vi "禹山pH_获取温度和测量值.vi"(8 "error in (no error)":errorcluster caption="错误输入（无错误）", 11 "MB_Serial session in":refnum<class "MB_Master_Serial.lvclass">) -> (0 "error out":errorcluster caption="错误输出", 2 "输出值":cluster{"温度测量值":sgl, "ORP":sgl, "pH":sgl}, 3 "MB_Serial session out":refnum<class "MB_Master_Serial.lvclass">)   [LabVIEW 2016, in "斯坦道多参数.lvlib"]
uses:
  <vilib>/Plasmionique/MB Master/MB_Master_Serial/MB_Master_Serial.lvclass
  C:/Program Files (x86)/National Instruments/LabVIEW 2016/vi.lib/Plasmionique/MB Master/MB_Master/MB_Master.lvclass
  <vilib>/Plasmionique/MB Master/MB Master.lvlib
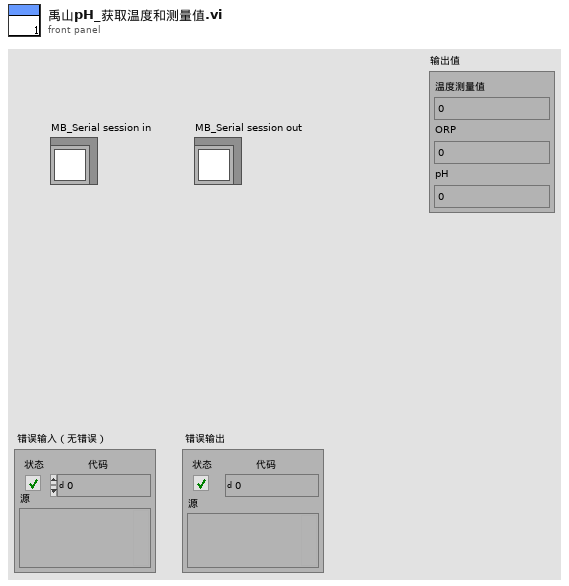
[diagram p1: front panel]
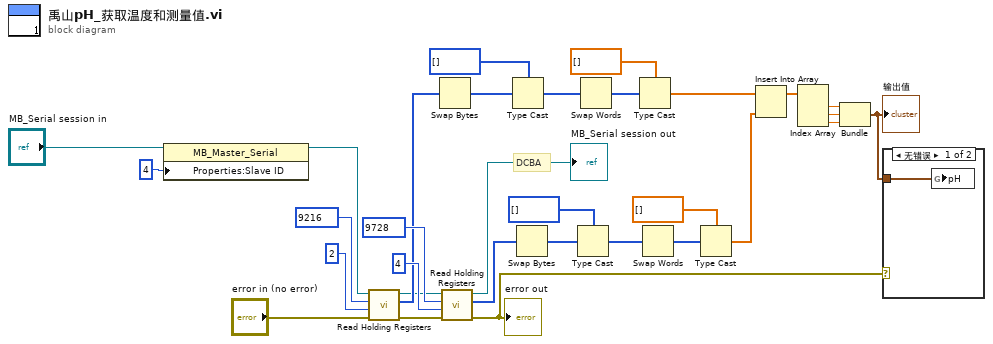
[diagram p0: block diagram]
diagram:
  # "DCBA"
  n1 = property class="MB_Master_Serial"(reference="MB_Serial session in", "Properties:Slave ID"=u16 4 ("y")) -> (reference out=w6:refnum<class "MB_Master_Serial.lvclass">)  [unwired: 1 in, 1 out]
  n2 = call <vilib>:"Read Holding Registers.vi"("error in (no error)"="error in (no error)", "quantity"=u16 2, "starting address"=u16 9216, "MB session in"=w6) -> ("error out"=w7:errorcluster, "Registers"=w11:u16[], "MB session out"=w5:refnum<class "MB_Master_Serial.lvclass">)  [unwired: 5 in]
  n3 = Swap Bytes(anything=w11) -> (byte swapped=w16:u16[])
  n4 = call <vilib>:"Read Holding Registers.vi"("error in (no error)"=w7, "quantity"=u16 4, "starting address"=u16 9728, "MB session in"=w5) -> ("error out"=w9:errorcluster, "Registers"=w23:u16[], "MB session out"=→"MB_Serial session out":refnum<class "MB_Master_Serial.lvclass">)  [unwired: 5 in]
  "error out" <- w9
  n5 = Type Cast(type=u32[] [] ("数组 2"), x=w16) -> (*(type *) &x=w14:u32[])
  n6 = Swap Bytes(anything=w23) -> (byte swapped=w22:u16[])
  n7 = Type Cast(type=u32[] [] ("数组 2"), x=w22) -> (*(type *) &x=w26:u32[])
  n8 = Swap Words(1:w14) -> (0:w12:u32[])
  n9 = Type Cast(type=sgl[] [] ("数组 2"), x=w12) -> (*(type *) &x=w4:sgl[])
  n10 = Swap Words(1:w26) -> (0:w28:u32[])
  n11 = Type Cast(type=sgl[] [] ("数组 2"), x=w28) -> (*(type *) &x=w2:sgl[])
  n12 = Insert Into Array(array=w4, new element=w2) -> (w3:sgl[])  [unwired: 1 in]
  n13 = Index Array(array=w3) -> (element #1=w21:sgl, element #2=w20:sgl, element #3=w1:sgl)  [unwired: 3 in]
  n14 = Bundle("数值"=w21, "数值"=w20, "数值"=w1) -> (w19:cluster{"数值":sgl, "数值":sgl, "数值":sgl})  [unwired: 1 in]
  "输出值" <- w19
  n15 = case shown="无错误" w9 {
    tunnel: w19 -> [w32 _]
    frame No Error {
      n16 = global write "禹山过程全局变量.vi" "pH"(w32) -> ()
    }
    frame Error {
    }
  }
